vi "Do Something Else and Wait for Reply.vi"(6 "wait for reply (T)":bool=TRUE, 8 "error in":errorcluster, 9 "X":dbl, 10 "Do Something Else Message":string) -> (0 "error out":errorcluster, 1 "timed out?":bool, 2 "Reply Payload":T1)   [LabVIEW 2022 SP3, in "MainPanel.lvlib"]
doc: "Send the Do Something Else request to the Module's Main.vi.\n_____\nBased on DQMH Project Template 7.0.1.1316."
uses:
  MainPanel.lvlib
  Do Something Else and Wait (Reply Payload)--cluster.ctl
  Do Something Else and Wait for Reply Argument--cluster.ctl
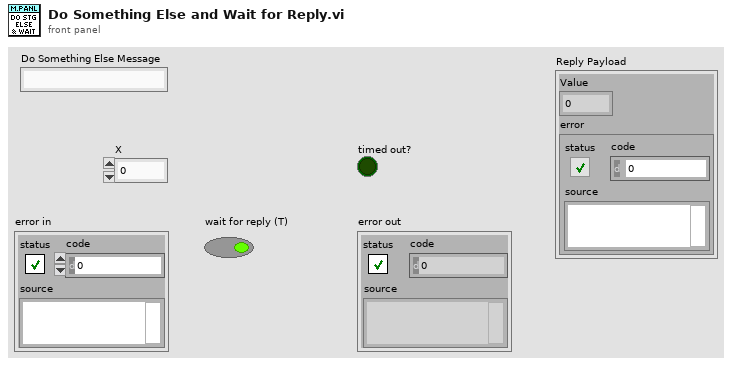
[diagram p1: front panel]
types:
  T1 = typedef "MainPanel.lvlib/Do Something Else and Wait (Reply Payload)--cluster.ctl" = cluster{"Value":dbl, "error":errorcluster}
  T2 = typedef "MainPanel.lvlib/Request Events--cluster.ctl" = cluster{"Stop Module":refnum<user-event>, "Do Something":refnum<user-event>, "Do Something Else":refnum<user-event>, "Do Something Else and Wait for Reply":refnum<user-event>, "Show Panel":refnum<user-event>, "Hide Panel":refnum<user-event>, "Get Module Execution Status":refnum<user-event>, "Show Diagram":refnum<user-event>, "Prepare":refnum<user-event>, "Configure":refnum<user-event>, "Request UI Display":refnum<user-event>}
  T3 = typedef "MainPanel.lvlib/Do Something Else and Wait for Reply Argument--cluster.ctl" = cluster{"Do Something Else Msg":string, "X":dbl, "Wait Notifier":refnum<notifier>, "wait for reply":bool}
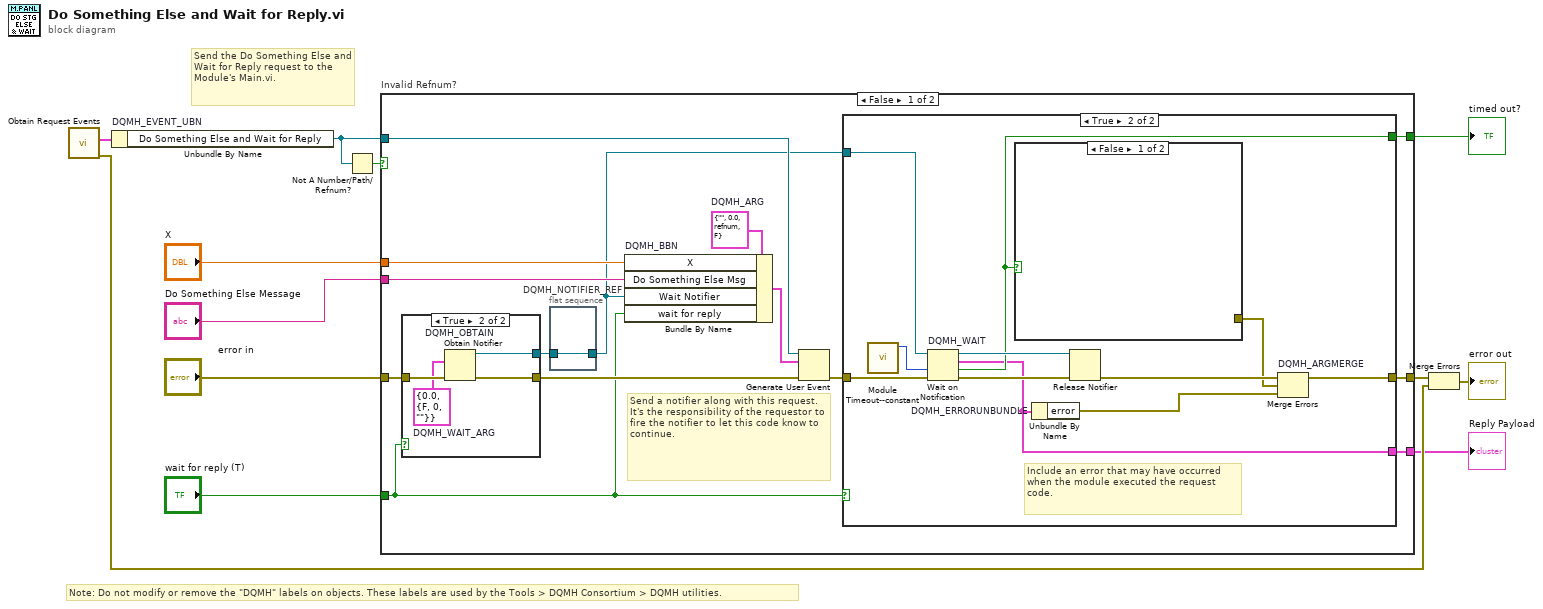
[diagram p0: block diagram]
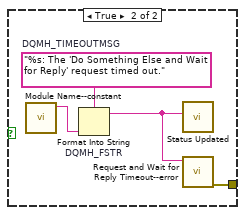
[diagram p3: hidden frame]
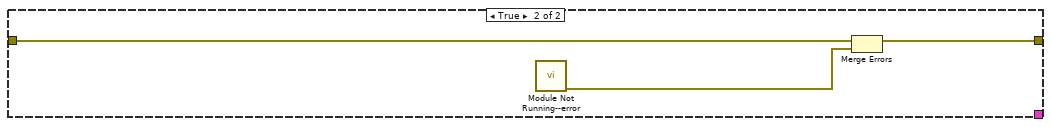
[diagram p5: hidden frame]
diagram:
  # "Note: Do not modify or remove the \"DQMH\" labels on objects. These labels are used by the Tools > DQMH Consortium > DQMH utilities."
  # "Send the Do Something Else and Wait for Reply request to the Module's Main.vi."
  n1 = call "Obtain Request Events.vi"() -> ("error out"=w11:errorcluster, "MainPanel Request Events"=w10:T2)  [unwired: 10 in]
  n2 = Unbundle By Name "DQMH_EVENT_UBN"(w10) -> ("Do Something Else and Wait for Reply"=w4:refnum<user-event>)
  n3 = Not A Number/Path/Refnum?(number/path/refnum=w4) -> (NaN/Path/Refnum?=w9:bool)
  n4 = case "Invalid Refnum?" shown="False" w9 {
    tunnel: [w17 w50] -> w5
    tunnel: "X" -> [w22 _]
    tunnel: "Do Something Else Message" -> [w21 _]
    tunnel: "error in" -> [w20 w49]
    tunnel: w4 -> [w19 _]
    tunnel: [w18 _] -> w3
    tunnel: [w16 _] -> w2
    tunnel: "wait for reply (T)" -> [w13 _]
    frame False {
      w25 = T3 {"Do Something Else Msg"="", "X"=0.0, "Wait Notifier"=refnum, "wait for reply"=FALSE}  # DQMH_ARG
      # "Send a notifier along with this request. It's the responsibility of the requestor to fire the notifier to let this code know to continue."
      n5 = case shown="True" w13 {
        tunnel: [w44 w48] -> w23
        tunnel: [_ w47] -> w15
        tunnel: w20 -> [w44 w46]
        frame False {
        }
        frame True {
          w45 = T1 {"Value"=0.0, "error"={"status"=FALSE, "code"=0, "source"=""}}  # DQMH_WAIT_ARG
          n6 = Obtain Notifier "DQMH_OBTAIN"(notification data type=w45, error in (no error)=w46) -> (notifier out=w47:refnum<notifier>, error out=w48:errorcluster)  [unwired: 2 in, 1 out]
        }
      }
      n7 = flat-sequence "DQMH_NOTIFIER_REF" {
        tunnel: w15 -> [w43]
        tunnel: [w43] -> w14
        frame #0 {
        }
      }
      n8 = Bundle By Name "DQMH_BBN"(cluster=w25, "X"=w22, "Do Something Else Msg"=w21, "Wait Notifier"=w14, "wait for reply"=w13) -> (w24:T3)
      n9 = Generate User Event(user event=w19, event data cluster=w24, error in=w23) -> (error out=w26:errorcluster)  [unwired: 1 in, 1 out]
      n10 = case shown="True" w13 {
        tunnel: w26 -> [w27 w38]
        tunnel: [_ w35] -> w18
        tunnel: [w27 w32] -> w17
        tunnel: [_ w31] -> w16
        tunnel: w14 -> [_ w30]
        frame False {
        }
        frame True {
          # "Include an error that may have occurred when the module executed the request code."
          n11 = call "Module Timeout--constant.vi"() -> ("Module Timeout"=w37:i32)  [unwired: 11 in]
          n12 = Wait on Notification "DQMH_WAIT"(notifier=w30, timeout in ms (-1)=w37, error in (no error)=w38) -> (notifier out=w36:refnum<notifier>, notification=w31:T1, timed out?=w35:bool, error out=w34:errorcluster)  [unwired: 1 in]
          n13 = case shown="False" w35 {
            tunnel: [_ w39] -> w28
            frame False {
            }
            frame True {
              w41 = "%s: The 'Do Something Else and Wait for Reply' request timed out."  # DQMH_TIMEOUTMSG
              n14 = call "Module Name--constant.vi"() -> ("Module Name"=w42:string)  [unwired: 11 in]
              n15 = Format Into String "DQMH_FSTR"(format string=w41, w42) -> (resulting string=w40:string)  [unwired: 2 in, 1 out]
              n16 = call "Status Updated.vi"("Status"=w40) -> ()  [unwired: 10 in, 1 out]
              n17 = call "Request and Wait for Reply Timeout--error.vi"("Error Message"=w40) -> ("error out"=w39:errorcluster)  [unwired: 10 in]
            }
          }
          n18 = Unbundle By Name "DQMH_ERRORUNBUNDLE"(w31) -> ("error"=w29:errorcluster)
          n19 = Release Notifier(notifier=w36, error in (no error)=w34) -> (error out=w33:errorcluster)  [unwired: 1 in, 2 out]
          n20 = Merge Errors "DQMH_ARGMERGE"(w33, w28, w29) -> (w32:errorcluster)
        }
      }
    }
    frame True {
      n21 = call "Module Not Running--error.vi"() -> ("error out"=w51:errorcluster)  [unwired: 11 in]
      n22 = Merge Errors(w49, w51) -> (w50:errorcluster)
    }
  }
  "timed out?" <- w3
  "Reply Payload" <- w2
  n23 = Merge Errors(w5, w11) -> (→"error out":errorcluster)
